vi "readTrigger.vi"(7 "address":string, 8 "error in (no error)":errorcluster) -> (0 "error out":errorcluster, 2 "Trigger":T1)   [LabVIEW 2016]
doc: "API to get the results of lockin calculation.\n\nIf address=\"\", this API reads from localhost\nIf address is remote lockin, you need to add this computer to allowed whitelist on the lockin computer you are trying to access."
uses:
  RemoteControl/Typedefs/PrivateEvents--LockinRemoteControl.setTrigger.ctl
  Instrument.Lockin/Typedefs/Instrument.Lockin.Commands--Enum.ctl
  RemoteControl/LockinRemoteControl.lvclass
  Instrument.Lockin/Instrument.Lockin.lvclass
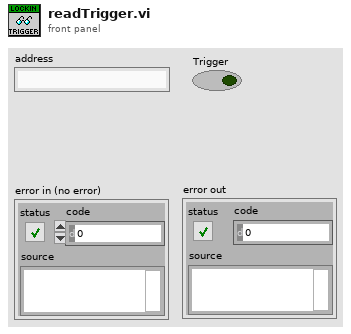
[diagram p1: front panel]
types:
  T1 = typedef "LockinRemoteControl.lvclass/PrivateEvents--LockinRemoteControl.setTrigger.ctl" = bool
  T2 = typedef "Instrument.Lockin.lvclass/Instrument.Lockin.Commands--Enum.ctl" = enum16{"configAO", "configREF", "configREFfilter", "configIVmode", "configRemote", "configReset", "configSampling", "assertTrigger", "getAO", "getAI", "getResults", "getTrigger", "getIVmode", "getSampling", "getAOconfig", "getREFconfig", "getREFfilter", "ACK", "UNK", "CLOSE", "configGain", "getGain"}
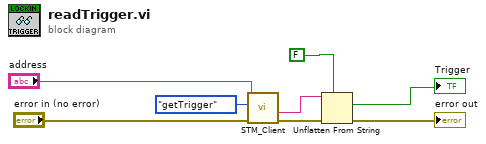
[diagram p0: block diagram]
diagram:
  n1 = call "STM_Client.vi"("error in (no error)"="error in (no error)", "Command"=Instrument.Lockin.Commands--Enum."getTrigger", "address"="address") -> ("error out"=w7:errorcluster, "data received from server"=w3:string)  [unwired: 7 in]
  n2 = Unflatten From String(type=T1 FALSE ("setTrigger"), binary string=w3, error in (no error)=w7) -> (value=→"Trigger":T1, error out=→"error out":errorcluster)  [unwired: 2 in, 1 out]
